vi "Call Function (Return Python Object).vi"(8 "error in (no error)":errorcluster, 9 "Arguments":T1[](array[typedef]), 10 "Function Name":string, 11 "Session Handle in":refnum<data-value>) -> (0 "error out":errorcluster, 1 "Returned Python Object Refnum":T1, 3 "Session Handle out":refnum<data-value>)   [LabVIEW 2020, in "G-Embedded-Python-Interpreter-Toolkit.lvlib"]
uses:
  G-Embedded-Python-Interpreter-Toolkit.lvlib
  Python Object Reference.ctl
  Python Object Type.ctl
  bin/gepit.cp310.32.dll
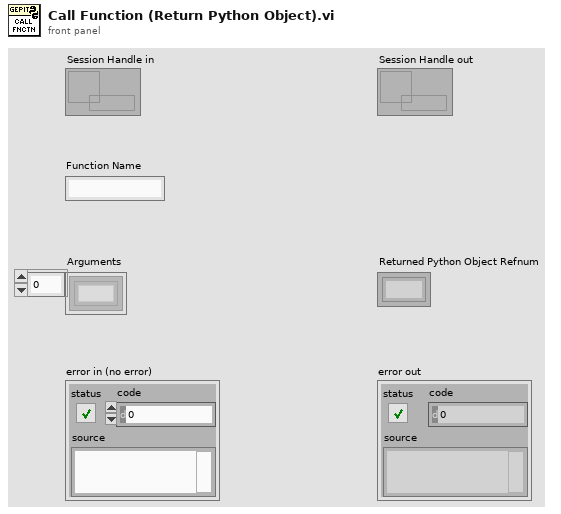
[diagram p1: front panel]
types:
  T1 = typedef "G-Embedded-Python-Interpreter-Toolkit.lvlib/Python Object Reference.ctl" = refnum<k1>
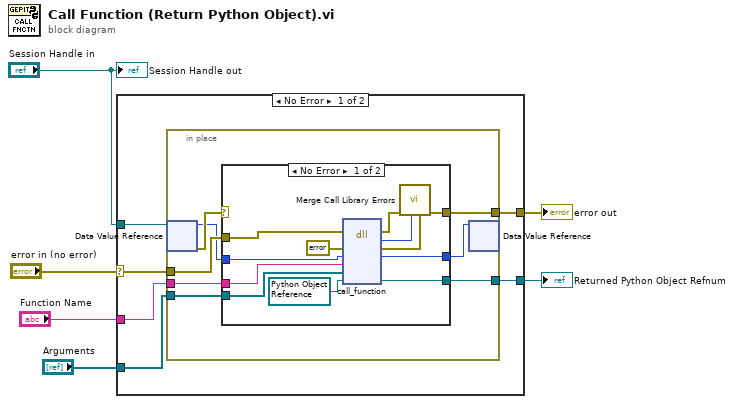
[diagram p0: block diagram]
diagram:
  n1 = case shown="No Error" "error in (no error)" {
    selector: "error in (no error)" -> [w11 w35]
    tunnel: "Session Handle in" -> [w12 _]
    tunnel: [w10 w35] -> w5
    tunnel: "Arguments" -> [w9 _]
    tunnel: [w8 _] -> w1
    tunnel: "Function Name" -> [w7 _]
    frame No Error {
      n2 = in-place {
        in-place-border: w11 -> [w19]
        in-place-border: [w16] -> w10
        in-place-border: w9 -> [w15]
        in-place-border: [w14] -> w8
        in-place-border: w7 -> [w13]
        n3 = in-place-dvr #1(w12) -> (w18:u64, w20:errorcluster)
        n4 = case shown="No Error" w20 {
          selector: w20 -> [_ w33]
          tunnel: w19 -> [w28 _]
          tunnel: w18 -> [w27 w34]
          tunnel: [w26 w34] -> w17
          tunnel: [w25 w33] -> w16
          tunnel: w15 -> [w22 _]
          tunnel: [w24 _] -> w14
          tunnel: w13 -> [w21 _]
          frame No Error {
            w23 = T1 refnum items=["PObj"] ("Returned Python Object Refnum")
            n5 = dll-call lib="C:/serenial/libraries/g-embedded-python-interpreter-toolkit/LabVIEW/bin/gepit.cp310.32.dll" fn="call_function"(error in=w28, "Error"=errorcluster {"status"=FALSE, "code"=0, "source"=""} ("error constant"), "Session"=w27, "Function Name"=w21, "Arguments"=w22, "Return"=w23) -> (error out=w31:errorcluster, "return type"=w30:i32, "Error"=w29:errorcluster, "Session"=w26:u64, "Return"=w24:T1)  [unwired: 4 in, 1 out]
            n6 = call "Merge Call Library Errors.vi"("Call Library Error"=w29, "Return Value"=w30, "error in"=w31) -> ("error out"=w25:errorcluster)  [unwired: 8 in]
          }
          frame Error {
          }
        }
        n7 = in-place-dvr #1(w17) -> ()  [unwired: 2 out]
      }
    }
    frame Error {
    }
  }
  "error out" <- w5
  "Returned Python Object Refnum" <- w1
  "Session Handle out" <- "Session Handle in"
